vi "Build Internal State String.vi"(2 "Seperator(<-)":string=" <- ", 5 "State":string, 7 "Arguments (\"\")":string, 9 "Additional Information":T1, 11 "Source (\"\")":string) -> (6 "State With Arguments":string)   [LabVIEW 2017, in "Communicable State Machine.lvlib"]
doc: "### Build Internal State String.vi\n\nConstruct a string containing JKI state machine states, arguments, and other information.\n\n-- <b>Controls</b> --\n- <b>State</b>: State string\n- <b>Arguments (\"\")</b>: Arguments for <b>State</b>\n- <b>Arg-State (\"\")</b>: State of the module sending this message at the time of sending\n- <b>Source (\"\")</b>: Name of the module sending this message\n\n-- <b>Indicators</b> --\n- <b>CSM Message String</b>: Concatenated CSM message string"
uses:
  Communicable State Machine.lvlib
  _Support/Typedef/_CSM_Response Source Message.ctl
  AdvanceAPI/CSM - Make String Arguments Safe.vi
  AdvanceAPI/CSM - Keywords.vi
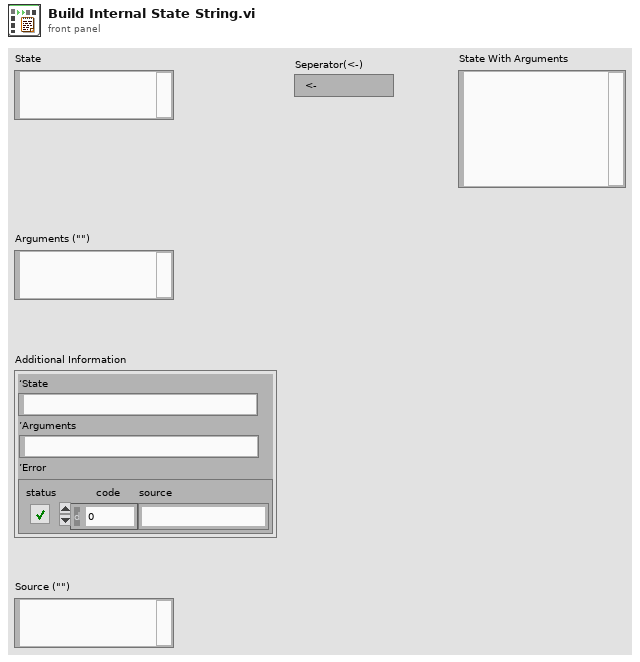
[diagram p1: front panel]
types:
  T1 = typedef "Communicable State Machine.lvlib/_CSM_Response Source Message.ctl" = cluster{"‘State":string, "’Arguments":string, "’Error":errorcluster}
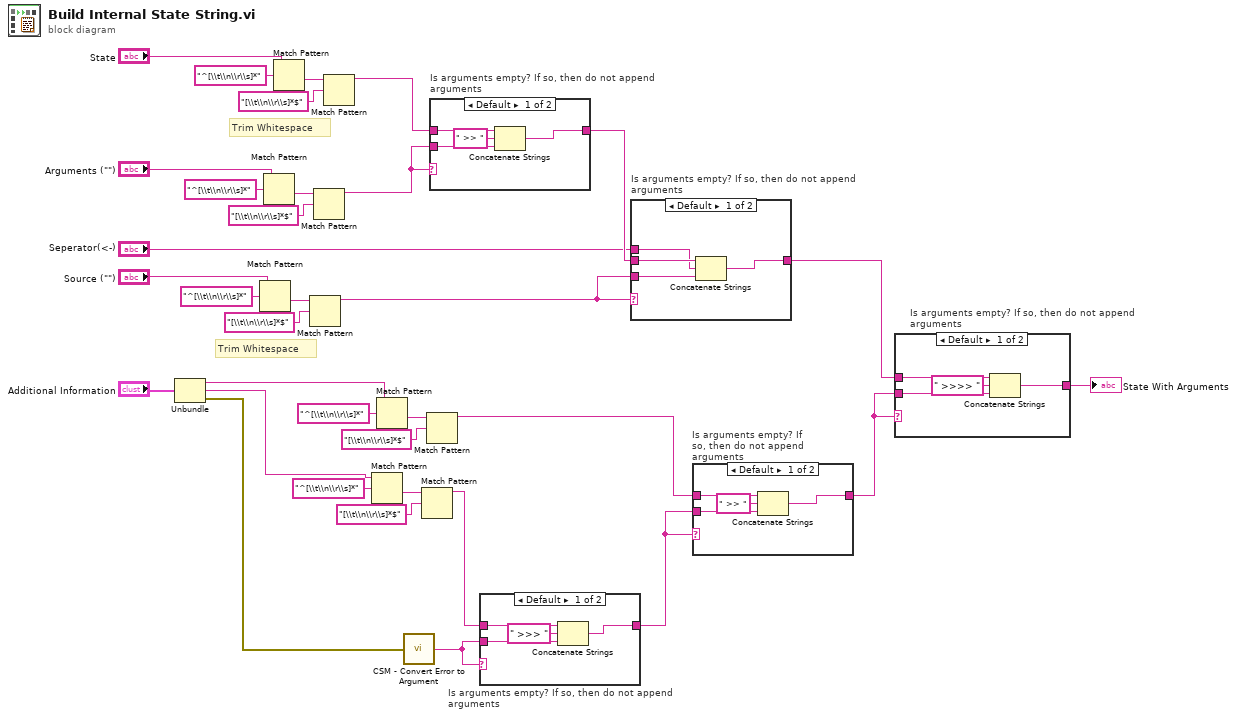
[diagram p0: block diagram]
diagram:
  # "Trim Whitespace"
  # "Trim Whitespace"
  n1 = Unbundle("Additional Information") -> ("‘State"=w12:string, "’Arguments"=w8:string, "’Error"=w6:errorcluster)
  n2 = Match Pattern(string="Source (\"\")", regular expression="^[\\t\\n\\r\\s]*") -> (after substring=w23:string)  [unwired: 1 in, 3 out]
  n3 = Match Pattern(string="Arguments (\"\")", regular expression="^[\\t\\n\\r\\s]*") -> (after substring=w28:string)  [unwired: 1 in, 3 out]
  n4 = Match Pattern(string="State", regular expression="^[\\t\\n\\r\\s]*") -> (after substring=w33:string)  [unwired: 1 in, 3 out]
  n5 = Match Pattern(string=w23, regular expression="[\\t\\n\\r\\s]*$") -> (before substring=w20:string)  [unwired: 1 in, 3 out]
  n6 = Match Pattern(string=w28, regular expression="[\\t\\n\\r\\s]*$") -> (before substring=w25:string)  [unwired: 1 in, 3 out]
  n7 = Match Pattern(string=w33, regular expression="[\\t\\n\\r\\s]*$") -> (before substring=w30:string)  [unwired: 1 in, 3 out]
  n8 = Match Pattern(string=w8, regular expression="^[\\t\\n\\r\\s]*") -> (after substring=w10:string)  [unwired: 1 in, 3 out]
  n9 = Match Pattern(string=w12, regular expression="^[\\t\\n\\r\\s]*") -> (after substring=w18:string)  [unwired: 1 in, 3 out]
  n10 = call "CSM - Convert Error to Argument.vi"("Error"=w6) -> ("Argument"=w5:string)  [unwired: 4 in]
  n11 = Match Pattern(string=w10, regular expression="[\\t\\n\\r\\s]*$") -> (before substring=w3:string)  [unwired: 1 in, 3 out]
  n12 = Match Pattern(string=w18, regular expression="[\\t\\n\\r\\s]*$") -> (before substring=w7:string)  [unwired: 1 in, 3 out]
  n13 = case "Is arguments empty? If so, then do not append arguments" shown="Default" w25 {
    tunnel: [w35 w39] -> w15
    tunnel: w30 -> [w38 w39]
    tunnel: w25 -> [w36 _]
    frame Default {
      n14 = Concatenate Strings(w38, " >> " ("string"), w36) -> (w35:string)
    }
    frame "" {
    }
  }
  n15 = case "Is arguments empty? If so, then do not append arguments" shown="Default" w5 {
    tunnel: [w40 w44] -> w2
    tunnel: w3 -> [w43 w44]
    tunnel: w5 -> [w41 _]
    frame Default {
      n16 = Concatenate Strings(w43, " >>> " ("string"), w41) -> (w40:string)
    }
    frame "" {
    }
  }
  n17 = case "Is arguments empty? If so, then do not append arguments" shown="Default" w20 {
    tunnel: [w46 w49] -> w14
    tunnel: w15 -> [w48 w49]
    tunnel: w20 -> [w47 _]
    tunnel: "Seperator(<-)" -> [w45 _]
    frame Default {
      n18 = Concatenate Strings(w48, w45, w47) -> (w46:string)
    }
    frame "" {
    }
  }
  n19 = case "Is arguments empty? If so, then do not append arguments" shown="Default" w2 {
    tunnel: [w50 w54] -> w4
    tunnel: w7 -> [w53 w54]
    tunnel: w2 -> [w51 _]
    frame Default {
      n20 = Concatenate Strings(w53, " >> " ("string"), w51) -> (w50:string)
    }
    frame "" {
    }
  }
  n21 = case "Is arguments empty? If so, then do not append arguments" shown="Default" w4 {
    tunnel: [w56 w59] -> w13
    tunnel: w14 -> [w58 w59]
    tunnel: w4 -> [w57 _]
    frame Default {
      n22 = Concatenate Strings(w58, " >>>> " ("string"), w57) -> (w56:string)
    }
    frame "" {
    }
  }
  "State With Arguments" <- w13
